vi "Filter vi.lib VIs.vi"(8 "Error In":errorcluster) -> (0 "Error Out":errorcluster)   [LabVIEW 2017, in "Tests.lvlib" / "Bookmark Manager.lvlib"]
uses:
  Bookmark Manager.lvlib
  <vilib>/addons/_JKI Toolkits/Caraya/classes/Test/Test.lvclass
  src/Bookmark Manager/Bookmark Manager.lvlib
  <vilib>/addons/_JKI Toolkits/Caraya/classes/Assert/Assert.lvclass
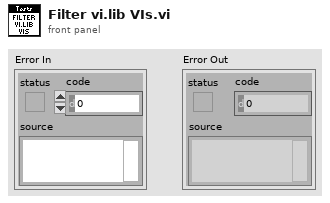
[diagram p1: front panel]
types:
  T1 = typedef "Bookmark Manager.lvlib/VI Information.ctl" = cluster{"App Info":T2, "Name":string, "Path":path}
  T2 = typedef "Bookmark Manager.lvlib/Application Information.ctl" = cluster{"Project":string, "Target":string}
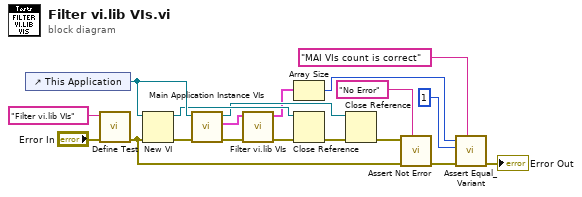
[diagram p0: block diagram]
diagram:
  n1 = control-ref of="This Application"() -> (w9:refnum<vi>)
  n2 = call <vilib>:"Define Test.vi"("error in (no error)"="Error In", "Label (VI Title)"="Filter vi.lib VIs") -> ("error out"=w11:errorcluster)  [unwired: 9 in]
  n3 = New VI(8:w11, 11:w9) -> (0:w10:errorcluster, 3:w7:refnum<vi>)  [unwired: 5 in]
  n4 = call "Main Application Instance VIs.vi"("Error In"=w10, "App In"=w9) -> ("Error Out"=w5:errorcluster, "VIs"=w3:T1[], "App Out"=w6:refnum<vi>)  [unwired: 7 in]
  n5 = call "Filter vi.lib VIs.vi"("Error In"=w5, "VIs In"=w3) -> ("Error Out"=w4:errorcluster, "VIs Out"=w2:T1[])  [unwired: 8 in]
  n6 = Array Size(array=w2) -> (size(s)=w1:i32)
  n7 = Close Reference(reference=w7, error in (no error)=w4) -> (error out=w8:errorcluster)
  n8 = Close Reference(reference=w6, error in (no error)=w8) -> (error out=w17:errorcluster)
  n9 = call <vilib>:"Assert Not Error.vi"("Label"="No Error", "error in (no error)"=w11, "Not Error?"=w17) -> ("error out"=w15:errorcluster)  [unwired: 8 in]
  n10 = call <vilib>:"Assert Equal_Variant.vi"("Label"="MAI VIs count is correct", "error in (no error)"=w15, "Y"=1, "X"=w1) -> ("error out"=→"Error Out":errorcluster)  [unwired: 7 in]
